vi "SetContactList.vi"(11 "recipients IN":string[](array[string])=["nmswyers@gmail.com"] caption="Errors & Warnings Email Recipients") -> (3 "recipients OUT":string[](array[string]))   [LabVIEW 2012]
panel:
  in  "recipients":string[](array[string])=["nmswyers@gmail.com"] caption="Errors & Warnings Email Recipients"
  in  "Cancel Button":bool
  in  "OK Button":bool
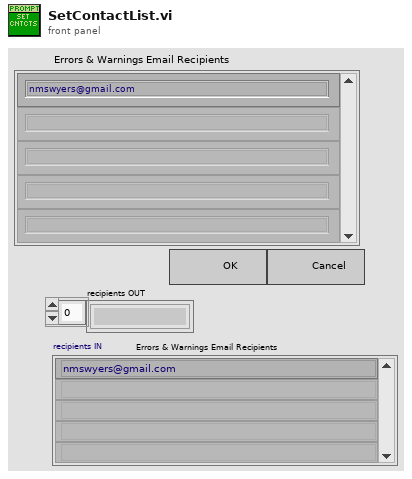
[diagram p1: front panel]
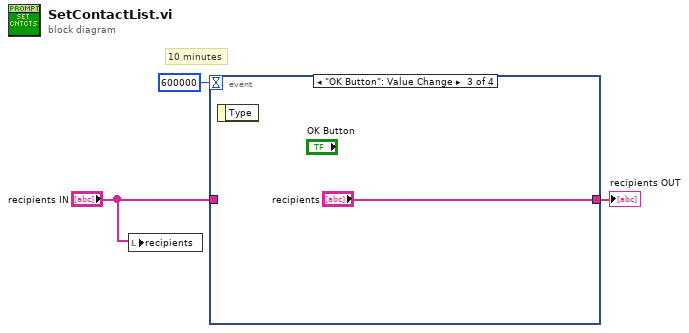
[diagram p0: block diagram]
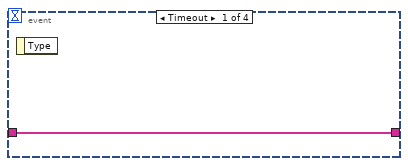
[diagram p2: hidden frame]
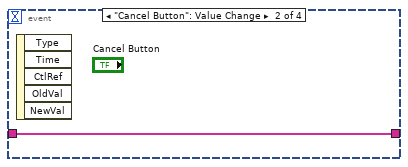
[diagram p3: hidden frame]
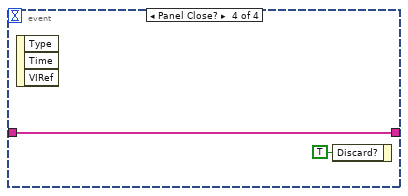
[diagram p4: hidden frame]
diagram:
  # "10 minutes"
  n1 = local write "recipients"("recipients IN") -> ()
  n2 = event shown="[2] \"OK Button\": Value Change" {
    selector: _ -> [_ _ _ _]
    dyn-events: _ -> [_ _ _ _]
    timeout: 600000 -> [_ _ _ _]
    tunnel: "recipients IN" -> [w4 w5 _ w7]
    tunnel: [w4 w5 "recipients" w7] -> w2
    event Timeout {
      n3 = event-data() -> ()  [unwired: 1 in, 1 out]
    }
    event "Cancel Button": Value Change {
      n4 = event-data() -> ()  [unwired: 1 in, 5 out]
    }
    event "OK Button": Value Change {
      n5 = event-data() -> ()  [unwired: 1 in, 1 out]
    }
    event Panel Close? {
      n6 = event-data() -> ()  [unwired: 1 in, 3 out]
      n7 = event-data("Discard?"=TRUE) -> ()  [unwired: 1 in, 1 out]
    }
  }
  "recipients OUT" <- w2
